vi "DP-Read IsoDP Data.vi"(0 "Path":path, 11 "error in (no error)":errorcluster) -> (4 "Freq":dbl[](array[numeric]), 6 "Criteria":dbl[](array[numeric]), 8 "Thresholds":dbl[][](array[numeric]), 15 "error out":errorcluster)   [LabVIEW 2020]
uses:
  <vilib>/regexp/Match Regular Expression.xnode
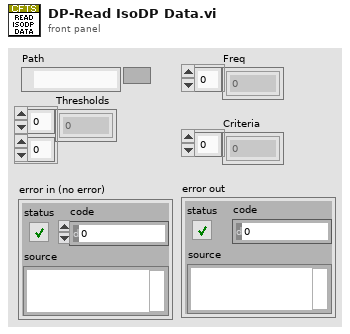
[diagram p1: front panel]
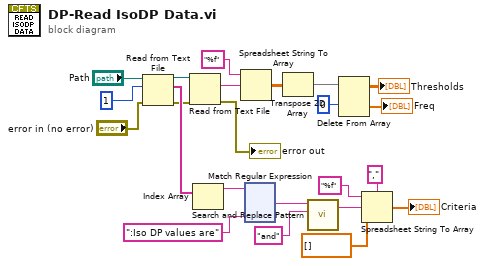
[diagram p0: block diagram]
diagram:
  n1 = Read from Text File(file (use dialog)="Path", count=1, error in="error in (no error)") -> (refnum out=w9:refnum<file>, text=w14:string[], error out=w8:errorcluster)  [unwired: 1 in, 1 out]
  n2 = Read from Text File(file (use dialog)=w9, error in=w8) -> (text=w10:string, error out=→"error out":errorcluster)  [unwired: 2 in, 2 out]
  n3 = Index Array(array=w14) -> (element=w15:string)  [unwired: 1 in]
  n4 = Spreadsheet String To Array(format string="%f", spreadsheet string=w10) -> (array=w11:dbl[][])  [unwired: 2 in]
  n5 = xnode "Match Regular Expression"("input string"=w15, "regular expression"=":Iso DP values are" ("search string/char (-)")) -> ("after match"=w17:string)  [unwired: 4 in, 4 out]
  n6 = Transpose 2D Array(2D array=w11) -> (transposed array=w4:dbl[][])
  n7 = call <vilib>:"Search and Replace Pattern.vi"("string"=w17, "regular expression (\"\")"="and" ("regular expression (\"\")")) -> ("result string"=w20:string)  [unwired: 3 in, 1 out]
  n8 = Delete From Array(array=w4, index (row)=0) -> (deleted portion=→"Freq":dbl[], array with subset deleted=→"Thresholds":dbl[][])  [unwired: 2 in]
  n9 = Spreadsheet String To Array(delimiter (Tab)=",", format string="%f", spreadsheet string=w20, array type (2D Dbl)=dbl[] []) -> (array=→"Criteria":dbl[])
